vi "writeBooleanFIFO.vi"(8 "error in (no error)":errorcluster, 9 "Timeout":i32, 10 "Data":bool[](array[boolean]), 11 "IWriteBooleanFIFO in":refnum<class "IWriteBooleanFIFO.lvclass">) -> (0 "error out":errorcluster, 2 "ElementsRemaining":u32, 3 "IWriteBooleanFIFO out":refnum<class "IWriteBooleanFIFO.lvclass">)   [LabVIEW 2015, in "RTFPGA.lvlib" / "IWriteBooleanFIFO.lvclass"]
uses:
  IWriteBooleanFIFO.lvclass
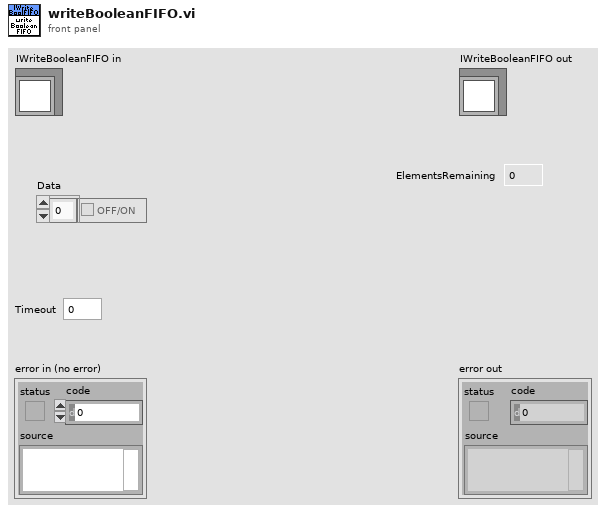
[diagram p1: front panel]
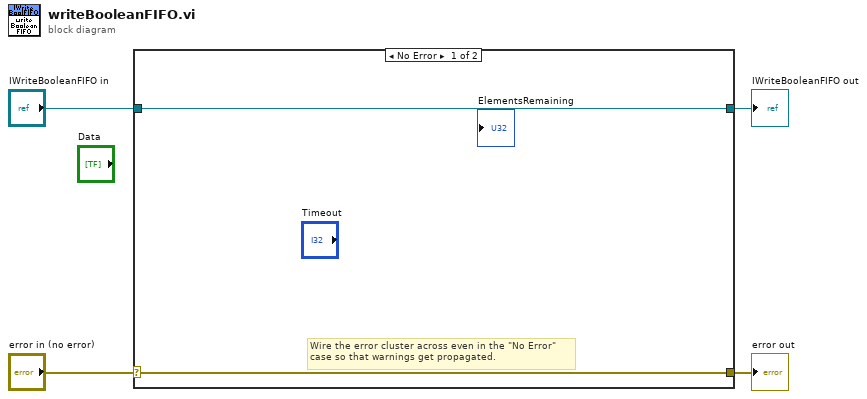
[diagram p0: block diagram]
diagram:
  n1 = case shown="No Error" "error in (no error)" {
    selector: "error in (no error)" -> [w5 w8]
    tunnel: [w5 w8] -> w3
    tunnel: [w6 w7] -> w1
    tunnel: "IWriteBooleanFIFO in" -> [w6 w7]
    frame No Error {
      # "Wire the error cluster across even in the \"No Error\"\ncase so that warnings get propagated."
    }
    frame Error {
    }
  }
  "error out" <- w3
  "IWriteBooleanFIFO out" <- w1
